vi "Get Section Names.vi"(8 "error in (no error)":errorcluster, 11 "refnum":T1) -> (0 "error out":errorcluster, 1 "section names":string[](array[string]), 3 "refnum out":T1)   [LabVIEW 2017, in "NI_LVConfig.lvlib"]
doc: "Gets the names of all sections from the configuration data identified by <B>refnum</B>."
uses:
  <vilib>/Utility/config.llb/NI_LVConfig.lvlib
  <vilib>/Utility/config.llb/Config Data RefNum.ctl
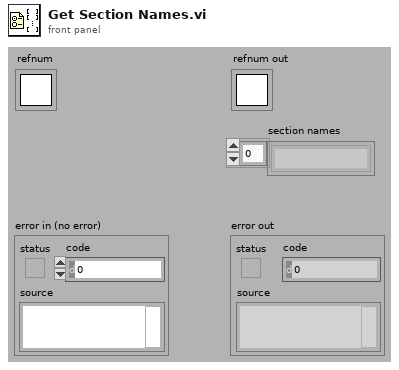
[diagram p1: front panel]
types:
  T1 = typedef "NI_LVConfig.lvlib/Config Data RefNum.ctl" = refnum<k1>
  T2 = typedef "NI_LVConfig.lvlib/Config Queue.ctl" = refnum<queue>
  T3 = typedef "NI_LVConfig.lvlib/Config Data.ctl" = cluster{"sections":T4[], "path":path, "dirty":bool}
  T4 = typedef "NI_LVConfig.lvlib/Section.ctl" = cluster{"name":string, "comment":string, "kvc":string[][]}
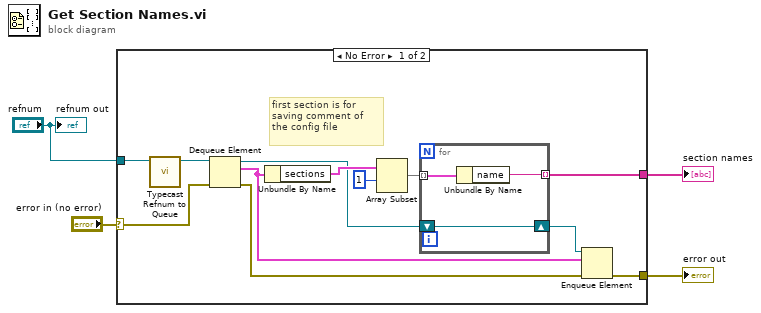
[diagram p0: block diagram]
diagram:
  n1 = case shown="No Error" "error in (no error)" {
    selector: "error in (no error)" -> [w10 w20]
    tunnel: [w15 _] -> w2
    tunnel: [w8 w20] -> w3
    tunnel: "refnum" -> [w14 _]
    frame No Error {
      # "first section is for saving comment of the config file"
      n2 = call <vilib>:"Typecast Refnum to Queue.vi"("refnum in"=w14) -> ("queue out"=w16:T2)  [unwired: 10 in]
      n3 = Dequeue Element(queue=w16, error in (no error)=w10) -> (queue out=w7:T2, element=w5:T3, error out=w9:errorcluster)  [unwired: 1 in, 1 out]
      n4 = Unbundle By Name(w5) -> ("sections"=w11:T4[])
      n5 = Array Subset(array=w11, index=1) -> (w12:T4[])  [unwired: 1 in]
      n6 = for {
        tunnel: w12 -> [w18] mode=indexing
        tunnel: [w19] -> w15 mode=indexing
        shift-right: [w17] -> w6
        shift-left: w7 -> [w17]
        n7 = Unbundle By Name(w18) -> ("name"=w19:string)
      }
      n8 = Enqueue Element(queue=w6, element=w5, error in (no error)=w9) -> (error out=w8:errorcluster)  [unwired: 1 in, 2 out]
    }
    frame Error {
    }
  }
  "error out" <- w3
  "section names" <- w2
  "refnum out" <- "refnum"
